vi "Configure Output List.vi"(7 "Source Mode  (0: Voltage)":u16(ring) items=["Voltage", "Current"], 8 "error in (no error)":errorcluster, 10 "Output List":dbl[](array[numeric]), 11 "VISA resource name":refnum<visa-resource-name>) -> (0 "error out":errorcluster, 3 "VISA resource name out":refnum<visa-resource-name>)   [LabVIEW 2012, in "Keithley 24XX.lvlib"]
doc: "Define a list of values for the source to output."
uses:
  Keithley 24XX.lvlib
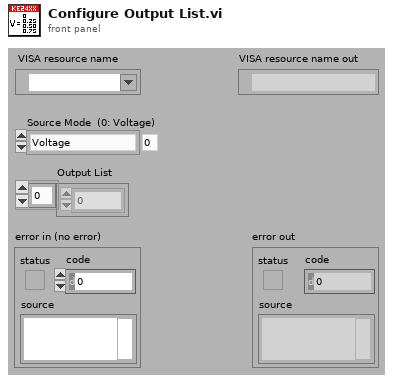
[diagram p1: front panel]
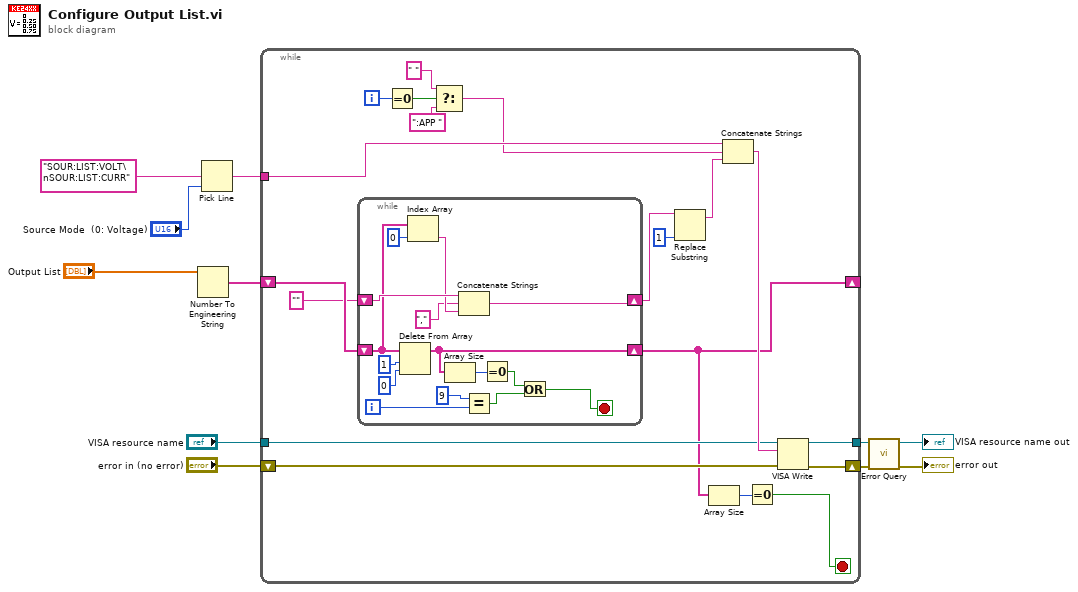
[diagram p0: block diagram]
diagram:
  n1 = Number To Engineering String(4:"Output List") -> (0:w6:string[])  [unwired: 3 in]
  n2 = Pick Line(multi-line string="SOUR:LIST:VOLT\nSOUR:LIST:CURR", line index="Source Mode  (0: Voltage)") -> (output string=w5:string)  [unwired: 1 in]
  n3 = while {
    tunnel: w5 -> [w24]
    tunnel: "VISA resource name" -> [w21]
    tunnel: [w19] -> w2
    shift-right: [w18] -> w1
    shift-left: "error in (no error)" -> [w20]
    shift-right: [w17] -> _
    shift-left: w6 -> [w30]
    i -> [w28]
    stop <- w15 stop-if-true
    n4 = while {
      shift-right: [w41] -> w13
      shift-left: "" -> [w44]
      shift-right: [w37] -> w17
      shift-left: w30 -> [w38]
      i -> [w35]
      stop <- w31 stop-if-true
      n5 = Delete From Array(array=w38, length=1, index=0) -> (array with subset deleted=w37:string[])  [unwired: 1 out]
      n6 = Index Array(array=w38, index=0) -> (element=w43:string)
      n7 = Array Size(array=w37) -> (size(s)=w36:i32)
      n8 = Concatenate Strings(w44, "," ("string"), w43) -> (w41:string)
      n9 = Equal?(x=9, y=w35) -> (x = y?=w33:bool)
      n10 = Equal To 0?(x=w36) -> (x = 0?=w32:bool)
      n11 = Or(x=w32, y=w33) -> (x .or. y?=w31:bool)
    }
    n12 = Equal To 0?(x=w28) -> (x = 0?=w27:bool)
    n13 = Select(t=" ", s=w27, f=":APP ") -> (s? t:f=w23:string)
    n14 = Replace Substring(2:1 ("length (len. of substring)"), 5:w13) -> (1:w12:string)  [unwired: 2 in, 1 out]
    n15 = Array Size(array=w17) -> (size(s)=w16:i32)
    n16 = Concatenate Strings(w24, w23, w12) -> (w22:string)
    n17 = Equal To 0?(x=w16) -> (x = 0?=w15:bool)
    n18 = VISA Write(VISA resource name=w21, write buffer=w22, error in (no error)=w20) -> (VISA resource name out=w19:refnum<visa-resource-name>, error out=w18:errorcluster)  [unwired: 1 out]
  }
  n19 = call "Error Query.vi"("error in (no error)"=w1, "VISA resource name"=w2) -> ("error out"=→"error out":errorcluster, "VISA resource name out"=→"VISA resource name out":refnum<visa-resource-name>)  [unwired: 6 in, 2 out]
